vi "AnOperation.vi"(8 "error in (no error)":errorcluster, 11 "Creator in":refnum<class "Creator.lvclass">) -> (0 "error out":errorcluster, 2 "ResultString":string, 3 "Creator out":refnum<class "Creator.lvclass">)   [LabVIEW 2020, in "FactoryMethod.lvlib" / "Creator.lvclass"]
uses:
  Creator.lvclass
  Creator.lvclass/Creator.ctl
  Private/Property/Product/Write Product.vi
  Product/Product.lvclass
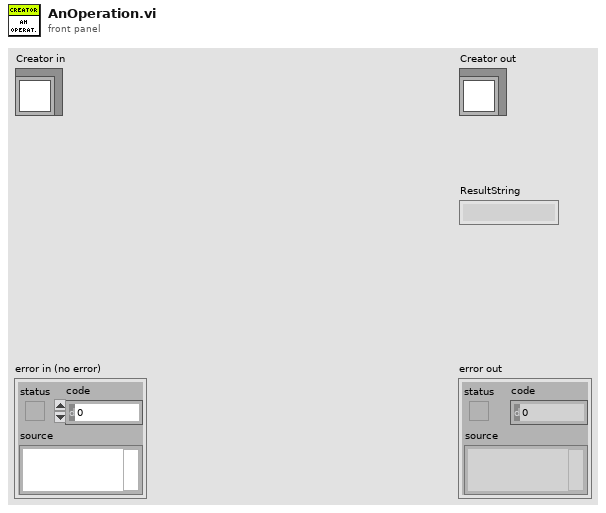
[diagram p1: front panel]
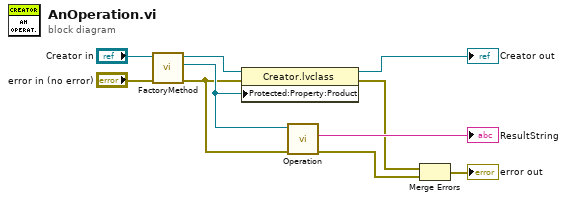
[diagram p0: block diagram]
diagram:
  n1 = call-dynamic "FactoryMethod.vi"("error in (no error)"="error in (no error)", "Creator in"="Creator in") -> ("error out"=w4:errorcluster, "Product."=w5:refnum<class "Product.lvclass">, "Creator out"=w7:refnum<class "Creator.lvclass">)  [unwired: 7 in]
  n2 = property class="Creator.lvclass"(reference=w7, error in=w4, "Protected:Property:Product"=w5) -> (reference out=→"Creator out":refnum<class "Creator.lvclass">, error out=w3:errorcluster)
  n3 = call-dynamic "Operation.vi"("error in (no error)"=w4, "Product in"=w5) -> ("error out"=w2:errorcluster, "ResultString"=→"ResultString":string)  [unwired: 7 in, 1 out]
  n4 = Merge Errors(w3, w2) -> (→"error out":errorcluster)
